vi "WaterLevel.vi"() -> ()   [LabVIEW 2017]
doc: "Printed Circuit Board Inspection\nDetermine whether PCB components are present and in the correct location using pattern matching. Match areas of inspection to a template of valid components. Use shift-invariant matching to inspect an oriented component (diode). Use rotation-invariant matching to inspect an unoriented component (resistor)."
uses:
  IMAQCV/IMAQCV.lvlib
  IMAQCV/LVOpenCV.lvlib
panel:
  in  "Image Delay ms":u32=5000
  out "Image":T1(plugin-control)
  out "Distance (Clamp (Rake) 1)":sgl format="%.2f"
  in  "Image File path":path=path "c:/vision/WaterLevel/001_01.jpg"
  out "Image Log path":path=path "c:/vision/Result.jpg"
  out "error out":errorcluster
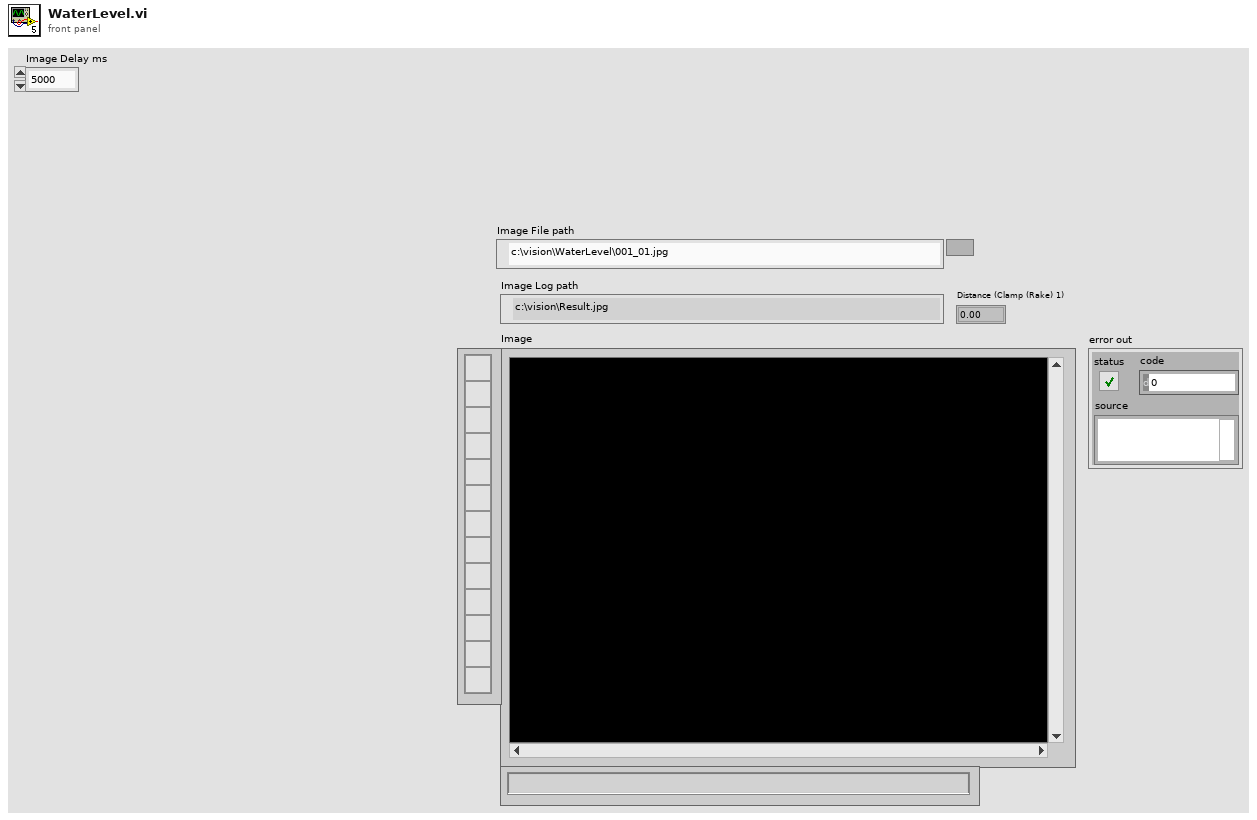
[diagram p1: front panel]
types:
  T1 = typedef "IMAQ Image.ctl" = refnum<image>
  T2 = cluster{"Desired Font (Application)":enum16{"User-specified Font", "Application Font", "System Font", "Dialog Font"}, "[User-specified Font]":cluster{"Font Name":string, "Size":i16, "Strikeout?":bool, "Italic?":bool, "Underline?":bool, "Outline?":bool, "Shadow?":bool, "Bold?":bool, "Rotation Angle":dbl}, "Horizontal Alignment":i16, "Vertical Alignment":i16}
  T3 = typedef "Image Type" = u32
  T4 = typedef "IMAQCV.lvlib/IMAQCV Image.ctl" = refnum<vi>
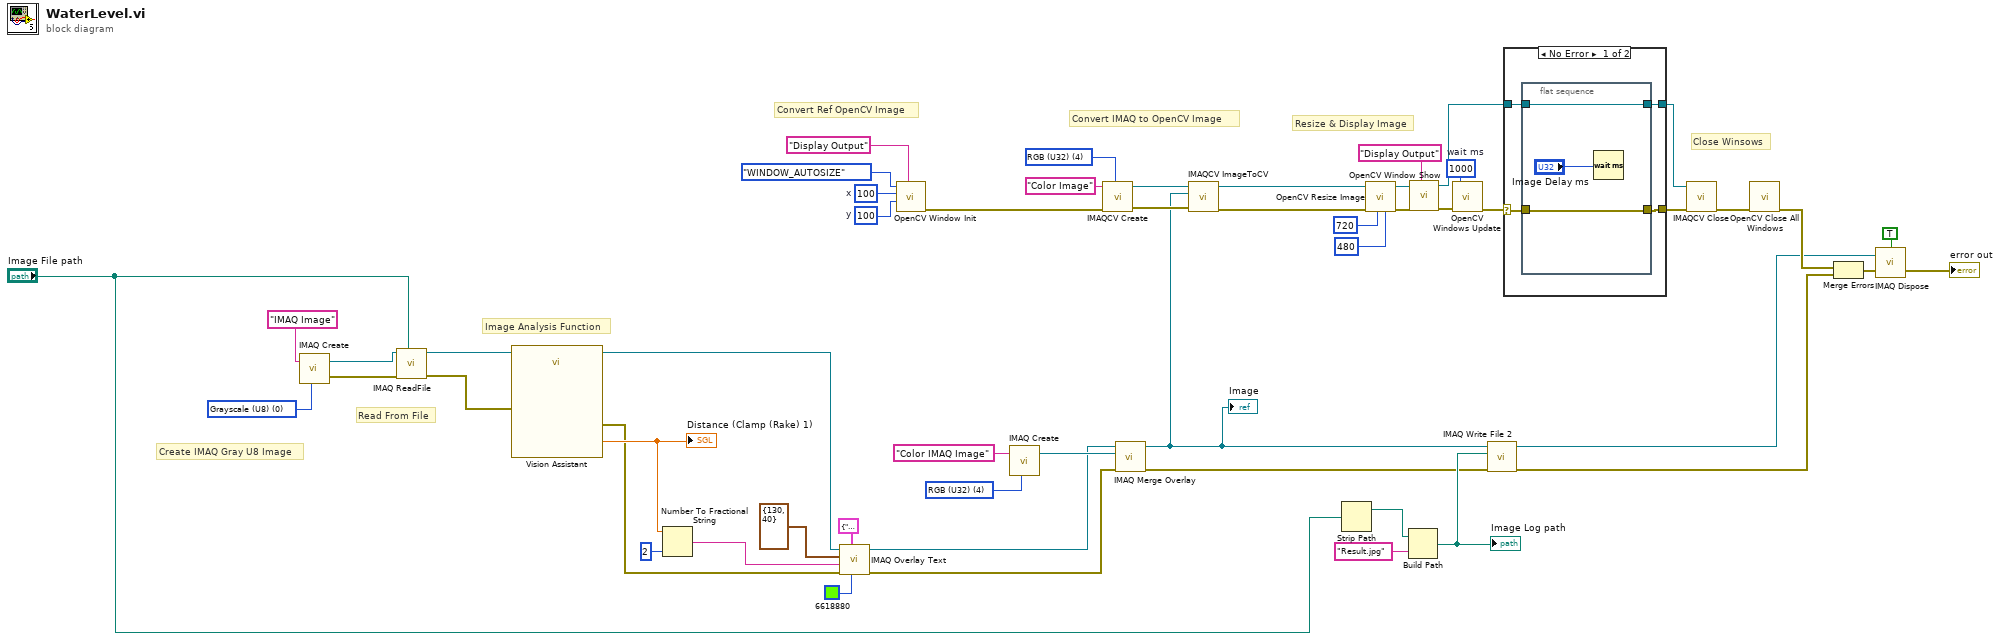
[diagram p0: block diagram]
diagram:
  w22 = 1000  # wait ms
  w29 = u32 100  # y
  w30 = u32 100  # x
  w33 = u32 4 items=["Grayscale (U8)", "Grayscale (I16)", "Grayscale (SGL)", "Complex (CSG)", "RGB (U32)", "HSL (U32)", "RGB (U64)", "Grayscale (U16)"] ("Image Type")
  w1 = T3 4 items=["Grayscale (U8)", "Grayscale (I16)", "Grayscale (SGL)", "Complex (CSG)", "RGB (U32)", "HSL (U32)", "RGB (U64)", "Grayscale (U16)"] ("Image Type")
  w4 = T3 0 items=["Grayscale (U8)", "Grayscale (I16)", "Grayscale (SGL)", "Complex (CSG)", "RGB (U32)", "HSL (U32)", "RGB (U64)", "Grayscale (U16)"] ("Image Type")
  # "Close Winsows"
  # "Resize & Display Image"
  # "Convert Ref OpenCV Image"
  # "Convert IMAQ to OpenCV Image"
  # "Image Analysis Function"
  # "Read From File"
  # "Create IMAQ Gray U8 Image"
  n1 = call "IMAQ Create"("Image Name"="IMAQ Image", "Image Type"=w4) -> ("New Image"=w53:T1, "error out"=w52:errorcluster)  [unwired: 2 in, 1 out]
  n2 = call "IMAQ ReadFile"("File Path"="Image File path", "error in (no error)"=w52, "Image"=w53) -> ("error out"=w5:errorcluster, "Image Out"=w44:T1)  [unwired: 2 in, 5 out]
  n3 = call "Vision Assistant"("Image In"=w44, "error in"=w5) -> ("Image Out"=w36:T1, "Distance (Clamp (Rake) 1)"=w42:sgl, "error out"=w3:errorcluster)  [unwired: 23 in]
  "Distance (Clamp (Rake) 1)" <- w42
  n4 = Number To Fractional String(number=w42, precision (6)=i16 2) -> (F-format string=w40:string)  [unwired: 2 in]
  n5 = call "IMAQ Overlay Text"("Text Color (black)"=u32 6618880, "Font, Size & Style"=T2 {"Desired Font (Application)"=enum."System Font", "[User-specified Font]"={"Font Name"="", "Size"=50, "Strikeout?"=FALSE, "Italic?"=FALSE, "Underline?"=FALSE, "Outline?"=FALSE, "Shadow?"=FALSE, "Bold?"=TRUE, "Rotation Angle"=0.0}, "Horizontal Alignment"=0, "Vertical Alignment"=0}, "error in (no error)"=w3, "String"=w40, "Origin"=cluster{"X":i32, "Y":i32} {"X"=130, "Y"=40}, "Image"=w36) -> ("error out"=w2:errorcluster, "Image Out"=w39:T1)  [unwired: 4 in]
  n6 = call "OpenCV Window Init.vi"("window name"="Display Output", "y"=w29, "x"=w30, "mode"=enum8{"WINDOW_AUTOSIZE", "WINDOW_FULLSCREEN"}."WINDOW_AUTOSIZE") -> ("error out"=w13:errorcluster)  [unwired: 7 in]
  n7 = call "IMAQ Create"("Image Name"="Color IMAQ Image", "Image Type"=w1) -> ("New Image"=w50:T1)  [unwired: 2 in, 2 out]
  n8 = call "IMAQCV Create.vi"("Image Type"=w33, "error in (no error)"=w13, "Image Name"="Color Image") -> ("error out"=w16:errorcluster, "Image Out"=w34:T4)  [unwired: 7 in]
  n9 = call "IMAQ Merge Overlay"("error in (no error)"=w2, "Image Dst"=w50, "Image Src"=w39) -> ("error out"=w45:errorcluster, "Image Dst Out"=w6:T1)  [unwired: 7 in]
  "Image" <- w6
  n10 = call "IMAQCV ImageToCV.vi"("error in (no error)"=w16, "Variant In"=w6, "CV in"=w34) -> ("error out"=w12:errorcluster, "CV out"=w21:T4)  [unwired: 7 in]
  n11 = Strip Path(path="Image File path") -> (stripped path=w48:path)  [unwired: 1 out]
  n12 = call "OpenCV Resize Image.vi"("height"=u32 480, "width"=u32 720, "error in (no error)"=w12, "image in"=w21) -> ("error out"=w25:errorcluster, "image out"=w26:T4)  [unwired: 6 in]
  n13 = Build Path(base path=w48, name or relative path="Result.jpg") -> (appended path=w46:path)
  "Image Log path" <- w46
  n14 = call "OpenCV Window Show.vi"("window name"="Display Output", "error in (no error)"=w25, "image in"=w26) -> ("error out"=w27:errorcluster, "image out"=w19:T4)  [unwired: 7 in]
  n15 = call "OpenCV Windows Update.vi"("error in (no error)"=w27, "wait ms"=w22) -> ("error out"=w15:errorcluster)  [unwired: 8 in, 1 out]
  n16 = call-poly "IMAQ Write File 2"("error in (no error)"=w45, "File Path"=w46, "Image"=w6) -> ("error out"=w8:errorcluster, "Image Out (duplicate)"=w9:T1)  [unwired: 7 in]
  n17 = case shown="No Error" w15 {
    selector: w15 -> [w55 w63]
    tunnel: [w58 w63] -> w20
    tunnel: w19 -> [w57 w62]
    tunnel: [w56 w62] -> w18
    frame No Error {
      n18 = flat-sequence {
        tunnel: [w61] -> w58
        tunnel: w55 -> [w61]
        tunnel: [w60] -> w56
        tunnel: w57 -> [w60]
        frame #0 {
          n19 = Wait (ms)(milliseconds to wait="Image Delay ms") -> ()  [unwired: 1 out]
        }
      }
    }
    frame Error {
    }
  }
  n20 = call "IMAQCV Close.vi"("error in (no error)"=w20, "Image"=w18) -> ("error out"=w17:errorcluster)  [unwired: 9 in]
  n21 = call "OpenCV Close All Windows.vi"("error in (no error)"=w17) -> ("error out"=w10:errorcluster)  [unwired: 10 in]
  n22 = Merge Errors(w10, w8) -> (w11:errorcluster)
  n23 = call "IMAQ Dispose"("All Images? (No)"=TRUE, "Image"=w9, "error in (no error)"=w11) -> ("error out"=→"error out":errorcluster)  [unwired: 3 in]
